vi "Set IsFrontMost.vi"(8 "error in (no error)":errorcluster, 10 "IsFrontMost":bool, 11 "ViewableActor in":refnum<class "ViewableActor.lvclass">) -> (0 "error out":errorcluster, 3 "ViewableActor out":refnum<class "ViewableActor.lvclass">)   [LabVIEW 2020, in "ViewableActor.lvlib" / "ViewableActor.lvclass"]
uses:
  ViewableActor.lvclass
  ViewableActor.lvclass/ViewableActor.ctl
  Read UI VI Ref.vi
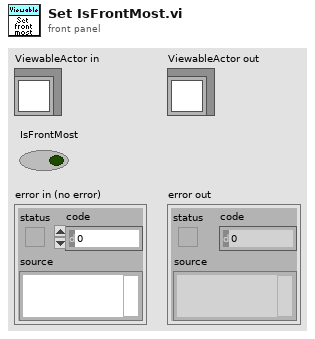
[diagram p1: front panel]
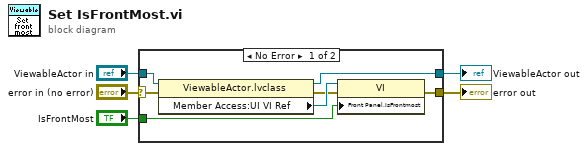
[diagram p0: block diagram]
diagram:
  n1 = case shown="No Error" "error in (no error)" {
    selector: "error in (no error)" -> [w7 w14]
    tunnel: [w6 w14] -> w4
    tunnel: [w11 w13] -> w2
    tunnel: "ViewableActor in" -> [w12 w13]
    tunnel: "IsFrontMost" -> [w9 _]
    frame No Error {
      n2 = property class="ViewableActor.lvclass"(reference=w12, error in=w7) -> (reference out=w11:refnum<class "ViewableActor.lvclass">, error out=w8:errorcluster, "Member Access:UI VI Ref"=w10:refnum<vi>)
      n3 = property class="VI"(reference=w10, error in=w8, "Front Panel.IsFrontmost"=w9) -> (error out=w6:errorcluster)  [unwired: 1 out]
    }
    frame Error {
    }
  }
  "error out" <- w4
  "ViewableActor out" <- w2
